vi "Record Period (global).vi"() -> ()   [LabVIEW 2019]
panel:
  in  "Record Period (ms)":u32
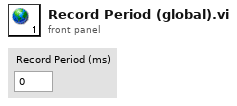
[diagram p1: front panel]
diagram:
